vi "Load VI on Subpanel.vi"(8 "error in (no error)":errorcluster, 10 "VI Refnum":refnum<vi>, 11 "Subpanel":refnum<vi>) -> (0 "error out":errorcluster)   [LabVIEW 2019, in "Panther Dashboard.lvlib"]
uses:
  Panther Dashboard.lvlib
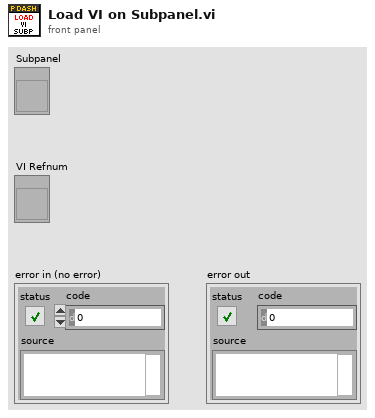
[diagram p1: front panel]
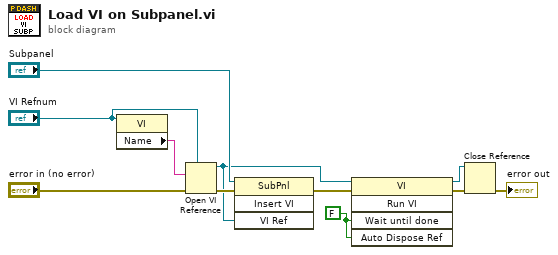
[diagram p0: block diagram]
diagram:
  w5 = FALSE ("Wait Until Done")
  n1 = property class="VI"(reference="VI Refnum") -> ("Name"=w8:string)  [unwired: 1 in, 2 out]
  n2 = Open VI Reference(type specifier VI Refnum (for type only)="VI Refnum", vi path=w8, error in (no error)="error in (no error)") -> (vi reference=w4:refnum<vi>, error out=w10:errorcluster)  [unwired: 3 in]
  n3 = invoke class="SubPnl" method="Insert VI"(reference="Subpanel", error in=w10, "VI Ref"=w4) -> (error out=w11:errorcluster)  [unwired: 1 in, 3 out]
  n4 = invoke class="VI" method="Run VI"(reference=w4, error in=w11, "Wait until done"=w5, "Auto Dispose Ref"=w5) -> (reference out=w6:refnum<vi>, error out=w9:errorcluster)  [unwired: 1 in, 3 out]
  n5 = Close Reference(reference=w6, error in (no error)=w9) -> (error out=→"error out":errorcluster)
